vi "CRYFFT CRYSoundLab complex.vi"(9 "dt":dbl=2.2675737e-05 format="%.7e", 10 "Window":i32(ring)=1 items=["None (Uniform)", "Hanning", "Hamming", "Blackman-Harris", "Exact Blackman", "Blackman", "Flat Top", "4 Term B-Harris", "7 Term B-Harris"], 11 "Time series":dbl[](array[numeric]) format="%.2f") -> (1 "window constants":cluster{"eq noise BW":dbl, "coherent gain":dbl} {"coherent gain" format="%.2f"; "eq noise BW" format="%.2f"}, 2 "df":dbl format="%.2f", 3 "Complex FFT (Vrms)":cdb[](array[numeric]) format="%.2f")   [LabVIEW 2013]
uses:
  <vilib>/Analysis/2dsp.llb/Real FFT.vi
  <vilib>/Analysis/0measdsp.llb/Scaled Time Domain Window (DBL).vi
  <vilib>/Analysis/NI_AALPro.lvlib
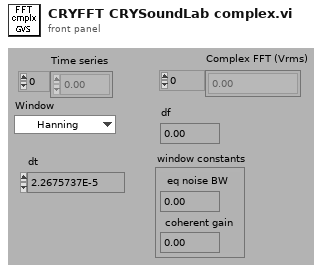
[diagram p1: front panel]
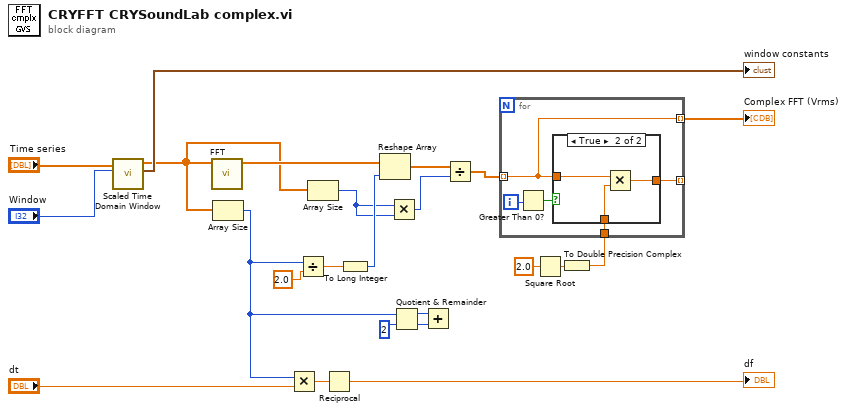
[diagram p0: block diagram]
diagram:
  n1 = call-poly <vilib>:"Scaled Time Domain Window.vi"("window"="Window", "X"="Time series") -> ("window properties"=→"window constants":cluster{"eq noise BW":dbl, "coherent gain":dbl}, "Windowed X"=w1:dbl[])  [unwired: 1 in, 7 out]
  n2 = call-poly <vilib>:"FFT.vi"("X"=w1) -> ("FFT {X}"=w9:cdb[])  [unwired: 2 in, 8 out]
  n3 = Array Size(array=w1) -> (size(s)=w8:i32)
  n4 = Multiply(x=w8, y="dt") -> (x*y=w20:dbl)
  n5 = Divide(x=w8, y=2.0) -> (x/y=w6:dbl)
  n6 = Array Size(array=w1) -> (size(s)=w4:i32)
  n7 = Reciprocal(x=w20) -> (1/x=→"df":dbl)
  n8 = To Long Integer(number=w6) -> (32bit integer=w5:i32)
  n9 = Reshape Array(w9, w5) -> (w11:cdb[])
  n10 = Multiply(x=w4, y=w4) -> (x*y=w3:i32)
  n11 = Quotient & Remainder(x=w8, y=2) -> (x-y*floor(x/y)=w14:i32, floor(x/y)=w13:i32)
  n12 = Add(x=w14, y=w13) -> ()  [unwired: 1 out]
  n13 = Divide(x=w11, y=w3) -> (x/y=w2:cdb[])
  n14 = Square Root(x=2.0) -> (sqrt(x)=w12:dbl)
  n15 = To Double Precision Complex(1:w12) -> (0:w16:cdb)
  n16 = for {
    tunnel: w2 -> [w24] mode=indexing
    tunnel: [w26] -> _ mode=indexing
    tunnel: w16 -> [w25]
    tunnel: [w24] -> w10 mode=indexing
    i -> [w28]
    n17 = Greater Than 0?(x=w28) -> (x > 0?=w27:bool)
    n18 = case shown="True" w27 {
      tunnel: [w29 w31] -> w26
      tunnel: w24 -> [w29 w32]
      tunnel: w25 -> [_ w30]
      frame False {
      }
      frame True {
        n19 = Multiply(x=w32, y=w30) -> (x*y=w31:cdb)
      }
    }
  }
  "Complex FFT (Vrms)" <- w10
